vi "Write mbed.lvclass.vi"(8 "error in (no error)":errorcluster, 10 "mbed.lvclass":refnum<class "mbed.lvclass">, 11 "DigitalOut in":refnum<class "DigitalOut.lvclass">) -> (0 "error out":errorcluster, 3 "DigitalOut out":refnum<class "DigitalOut.lvclass">)   [LabVIEW 2009, in "DigitalOut.lvclass"]
uses:
  DigitalOut.lvclass
  mbed.lvclass
  DigitalOut.lvclass/DigitalOut.ctl
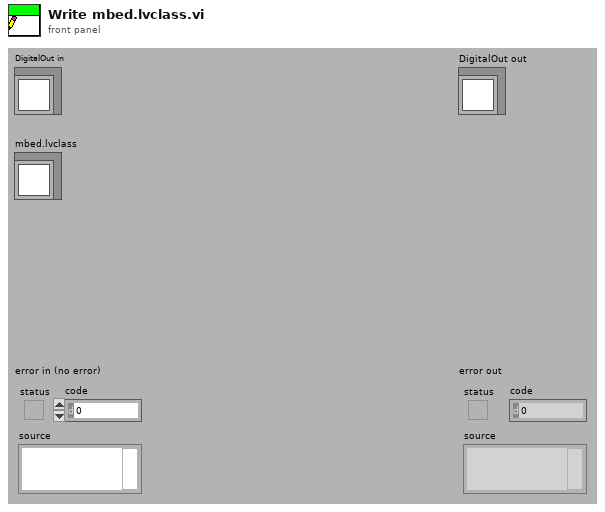
[diagram p1: front panel]
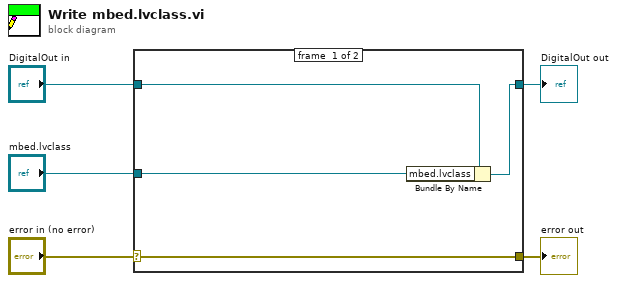
[diagram p0: block diagram]
diagram:
  n1 = case shown="No Error" "error in (no error)" {
    selector: "error in (no error)" -> [w9 w10]
    tunnel: [w9 w10] -> w4
    tunnel: [w7 w11] -> w2
    tunnel: "DigitalOut in" -> [w8 w11]
    tunnel: "mbed.lvclass" -> [w6 _]
    frame #0 {
      n2 = Bundle By Name(cluster=w8, "mbed.lvclass"=w6) -> (w7:refnum<class "DigitalOut.lvclass">)
    }
    frame #1 {
    }
  }
  "error out" <- w4
  "DigitalOut out" <- w2
